vi "Format Extension.vi"(3 "Format":T1) -> (1 "Extension":string)   [LabVIEW 2020, in "VolatusConfig.lvlib"]
uses:
  VolatusConfig.lvlib
  Config Format.ctl
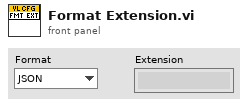
[diagram p1: front panel]
types:
  T1 = typedef "VolatusConfig.lvlib/Config Format.ctl" = enum16{"JSON", "INI", "SQLite"}
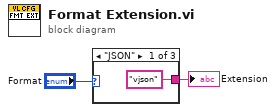
[diagram p0: block diagram]
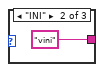
[diagram p2: hidden frame]
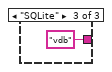
[diagram p3: hidden frame]
diagram:
  n1 = case shown="\"JSON\"" "Format" {
    tunnel: ["vjson" "vini" "vdb"] -> w1
    frame "JSON" {
    }
    frame "INI" {
    }
    frame "SQLite" {
    }
  }
  "Extension" <- w1
